vi "Conveyer Belt Set.vi"(0 "Conveyer Belt Info":T1) -> ()   [LabVIEW 2012]
uses:
  Conveyer Belt Global Data.vi
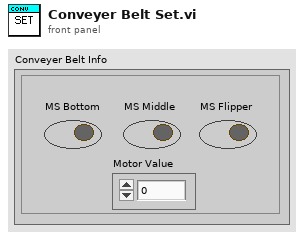
[diagram p1: front panel]
types:
  T1 = cluster{"MS Bottom":bool, "MS Middle":bool, "MS Flipper":bool, "Motor Value":dbl}
  T2 = typedef "WPI_MotorControlDeviceRef.ctl" = cluster{"DeviceStatus":errorcluster, "Type":enum16{"PWM", "CAN"}, "PWM":cluster{"Digital Module":T3, "PWM Channel":T4, "DeadBand":T5}, "CAN":cluster{"Device Number":u8, "Control Mode":T6, "Semaphore":T7, "Max Vout":dbl}, "Invert":bool, "TransformRef":T8, "InvTransformRef":T8}
  T3 = typedef "FPGA_TypedefDigitalModule.ctl" = enum16{"Digital Module 1", "Digital Module 2"}
  T4 = typedef "FPGA_DIOPWMChannel.ctl" = enum8{"PWM 1", "PWM 2", "PWM 3", "PWM 4", "PWM 5", "PWM 6", "PWM 7", "PWM 8", "PWM 9", "PWM 10", "Invalid"}
  T5 = typedef "WPI_PWMDeadband.ctl" = cluster{"Name":string, "maxPositivePwm":i32, "minPositivePwm":i32, "centerPwm":i32, "maxNegativePwm":i32, "minNegativePwm":i32, "angularRange":u16}
  T6 = typedef "WPI_CANJaguar_ControlMode.ctl" = enum8{"Percent VBus", "Current", "Speed", "Position", "Voltage"}
  T7 = typedef "Semaphore RefNum" = refnum<k1>
  T8 = typedef "WPI_PWMTransform_ConPane.ctl" = refnum<vi>
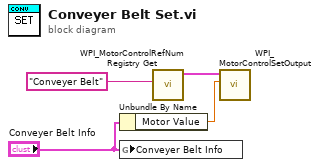
[diagram p0: block diagram]
diagram:
  n1 = Unbundle By Name("Conveyer Belt Info") -> ("Motor Value"=w3:dbl)
  n2 = global write "Conveyer Belt Global Data.vi" "Conveyer Belt Info"("Conveyer Belt Info") -> ()
  n3 = call <vilib>:"WPI_MotorControlRefNum Registry Get.vi"("refnum name"="Conveyer Belt") -> ("MotorControlDevRef"=w2:T2)  [unwired: 9 in, 1 out]
  n4 = call <vilib>:"WPI_MotorControlSetOutput.vi"("Output"=w3, "MotorControlDevRef"=w2) -> ()  [unwired: 7 in, 3 out]
